vi "Read List Of Kaslis in this Schedule.vi"(8 "error in (no error)":errorcluster, 11 "Schedule in":refnum<class "Schedule.lvclass">) -> (0 "error out":errorcluster, 2 "List of FPGAs":set{string}(c389), 3 "Schedule out":refnum<class "Schedule.lvclass">)   [LabVIEW 2020, in "Run Utilities.lvlib" / "Schedule.lvclass"]
doc: "Go over the entire schedule and create a list of Kaslis that are used."
uses:
  Schedule.lvclass
  Schedule.lvclass/Schedule.ctl
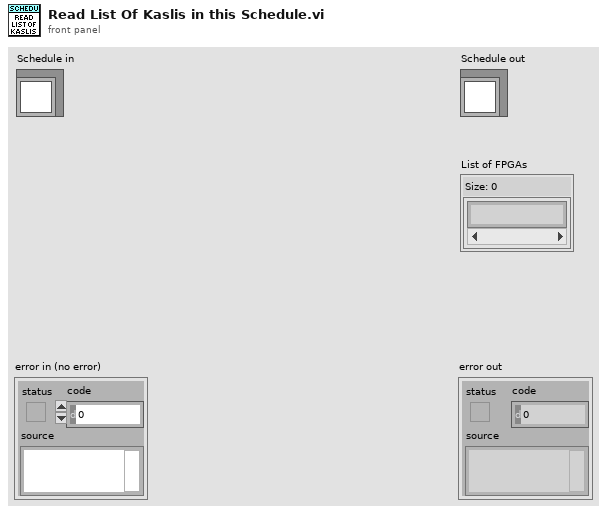
[diagram p1: front panel]
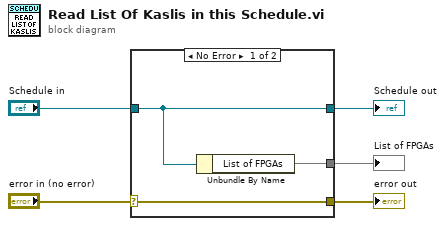
[diagram p0: block diagram]
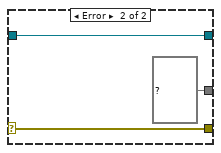
[diagram p2: hidden frame]
diagram:
  n1 = case shown="No Error" "error in (no error)" {
    selector: "error in (no error)" -> [w6 w11]
    tunnel: [w6 w11] -> w4
    tunnel: [w8 w10] -> w2
    tunnel: "Schedule in" -> [w8 w10]
    tunnel: [w7 set{string} {} ("List of FPGAs")] -> w1
    frame No Error {
      n2 = Unbundle By Name(w8) -> ("List of FPGAs"=w7:set{string})
    }
    frame Error {
    }
  }
  "error out" <- w4
  "Schedule out" <- w2
  "List of FPGAs" <- w1
